vi "Launch Module.vi"(11 "Error in":errorcluster caption="Error in (no error)") -> (15 "Error out":errorcluster)   [LabVIEW 2019]
doc: "<Developer>\nGPower\n21/9 2019"
uses:
  <vilib>/GPower/Actor/Library/Actor Class/Actor.lvclass
  Module.lvclass
  <vilib>/GPower/Logger - MCL/Library/MCL Logger Class/MCL Logger.lvclass
  <vilib>/GPower/Actor/Library/Actor Interface Class/Actor Interface.lvclass
  <vilib>/GPower/Actor/Library/Final Message Class/Final Message.lvclass
  <vilib>/GPower/Actor/Library/Final Message Class/Accessors/Decode Final Message (No Cast).vi
  <vilib>/GPower/Message/Library/Message Class/Message.lvclass
  C:/Program Files (x86)/National Instruments/LabVIEW 2019/vi.lib/GPower/Actor/Library/Actor Class/Actor.lvclass
  C:/Program Files (x86)/National Instruments/LabVIEW 2019/vi.lib/GPower/Logger/Library/Logger Class/Logger.lvclass
panel:
  in  "Multicolumn Listbox":i32(listbox)
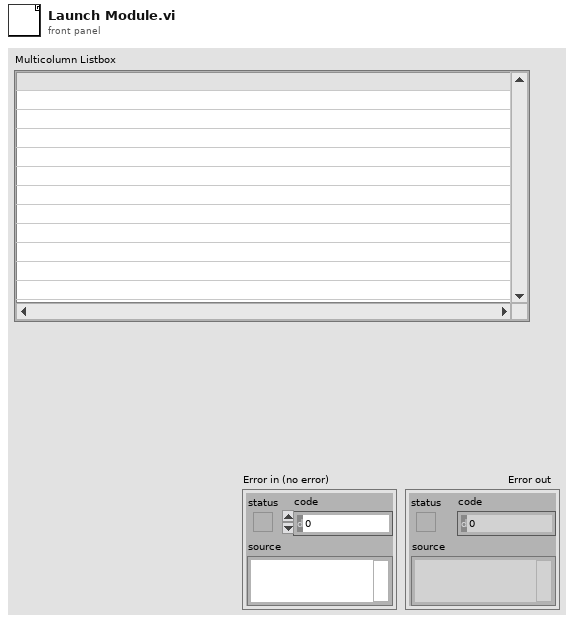
[diagram p1: front panel]
types:
  T1 = typedef "GP Actor.lvlib/Actor Interface.lvclass/Registered Actor Events.ctl" = cluster{"Actor Messages":refnum<event-registration>, "Actor Stopped":refnum<event-registration>, "Actor Stop":refnum<event-registration>}
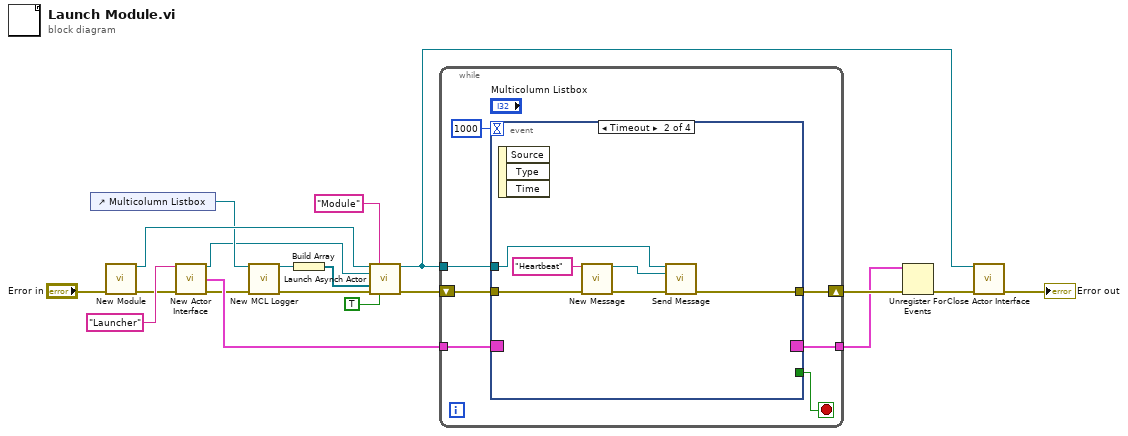
[diagram p0: block diagram]
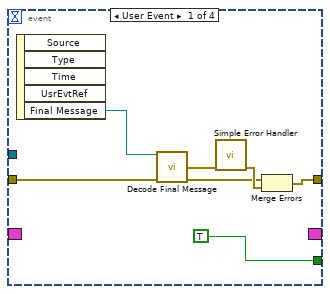
[diagram p2: hidden frame]
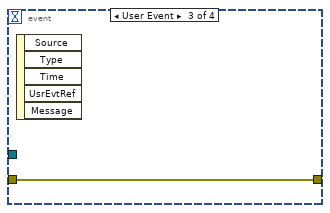
[diagram p3: hidden frame]
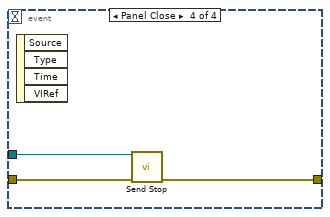
[diagram p4: hidden frame]
diagram:
  n1 = control-ref of="Multicolumn Listbox"() -> (w16:refnum<vi>)
  n2 = call "New Module.vi"("Error in"="Error in") -> ("New Module"=w19:refnum<class "Module.lvclass">, "Error out"=w2:errorcluster)  [unwired: 13 in]
  n3 = call <vilib>:"New Actor Interface.vi"("My Name"="Launcher", "Error in"=w2) -> ("New Actor Interface"=w11:refnum<class "Actor Interface.lvclass">, "Registered Actor Events"=w10:T1, "Error out"=w9:errorcluster)  [unwired: 11 in]
  n4 = call <vilib>:"New MCL Logger.vi"("Multicolumn Listbox"=w16, "Error in"=w9) -> ("MCL Logger"=w15:refnum<class "MCL Logger.lvclass">, "Error out"=w8:errorcluster)  [unwired: 12 in]
  n5 = Build Array(w15) -> (w14:refnum<class "MCL Logger.lvclass">[])
  n6 = call <vilib>:"Launch Asynch Actor.vi"("Actor"=w19, "Actor Name"="Module", "Caller Interface"=w11, "Loggers"=w14, "Error in"=w8, "Expect Self Stop?"=TRUE) -> ("Actor Interface"=w3:refnum<class "Actor Interface.lvclass">, "Error out"=w13:errorcluster)  [unwired: 8 in]
  n7 = while {
    shift-right: [w25] -> w7
    shift-left: w13 -> [w26]
    tunnel: w3 -> [w22]
    tunnel: w10 -> [w24]
    tunnel: [w23] -> w6
    stop <- w21 stop-if-true
    n8 = event shown="[1] Timeout" {
      selector: w24 -> [_ _ _ _]
      dyn-events: [_ _ _ _] -> w23
      timeout: 1000 -> [_ _ _ _]
      tunnel: w26 -> [w33 w37 w40 w43]
      tunnel: [w28 w39 w40 w41] -> w25
      tunnel: w22 -> [_ w38 _ w42]
      tunnel: [TRUE _ _ _] -> w21
      event User Event {
        n9 = event-data() -> ("Final Message"=w32:refnum<class "Final Message.lvclass">)  [unwired: 1 in, 4 out]
        n10 = call-poly <vilib>:"Decode Final Message.vi"("Final Message in"=w32, "Error in"=w33) -> ("Actor Final Error"=w31:errorcluster, "Error out"=w29:errorcluster)  [unwired: 9 in, 3 out]
        n11 = call <vilib>:"Simple Error Handler.vi"("error in (no error)"=w31) -> ("error out"=w30:errorcluster)  [unwired: 4 in, 4 out]
        n12 = Merge Errors(w29, w30) -> (w28:errorcluster)
      }
      event Timeout {
        n13 = event-data() -> ()  [unwired: 1 in, 3 out]
        n14 = call <vilib>:"New Message.vi"("Name"="Heartbeat", "Error in"=w37) -> ("New Message"=w35:refnum<class "Message.lvclass">, "Error out"=w36:errorcluster)  [unwired: 12 in]
        n15 = call <vilib>:"Send Message.vi"("Receiver"=w38, "Message"=w35, "error in (no error)"=w36) -> ("error out"=w39:errorcluster)  [unwired: 12 in]
      }
      event User Event {
        n16 = event-data() -> ()  [unwired: 1 in, 5 out]
      }
      event Panel Close {
        n17 = event-data() -> ()  [unwired: 1 in, 4 out]
        n18 = call <vilib>:"Send Stop.vi"("Receiver"=w42, "Error in"=w43) -> ("Error out"=w41:errorcluster)  [unwired: 13 in]
      }
    }
  }
  n19 = Unregister For Events(event registration refnum=w6, error in=w7) -> (error out=w5:errorcluster)
  n20 = call <vilib>:"Close Actor Interface.vi"("Actor Interface"=w3, "Error in"=w5) -> ("Error out"=→"Error out":errorcluster)  [unwired: 13 in]
